vi "写入检测值.vi"(8 "error in (no error)":errorcluster caption="错误输入（无错误）", 10 "检测值":sgl, 11 "DGUS输入":refnum<class "DGUS.lvclass">) -> (0 "error out":errorcluster caption="错误输出", 3 "DGUS输出":refnum<class "DGUS.lvclass">)   [LabVIEW 2016, in "DGUS.lvlib" / "DGUS.lvclass"]
uses:
  DGUS.lvclass
  DGUS.lvclass/DGUS.ctl
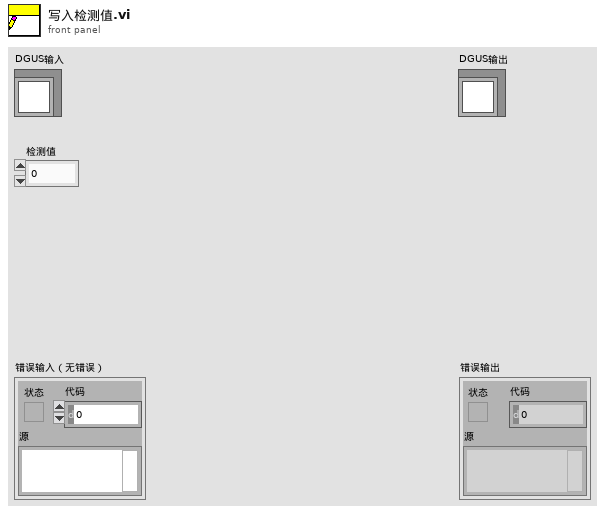
[diagram p1: front panel]
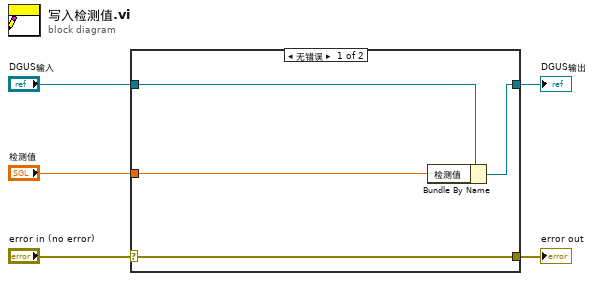
[diagram p0: block diagram]
diagram:
  n1 = case shown="无错误" "error in (no error)" {
    selector: "error in (no error)" -> [w9 w10]
    tunnel: [w9 w10] -> w4
    tunnel: [w7 w11] -> w2
    tunnel: "DGUS输入" -> [w8 w11]
    tunnel: "检测值" -> [w6 _]
    frame No Error {
      n2 = Bundle By Name(cluster=w8, "检测值"=w6) -> (w7:refnum<class "DGUS.lvclass">)
    }
    frame Error {
    }
  }
  "error out" <- w4
  "DGUS输出" <- w2
